vi "Speed.vi"(8 "error in":errorcluster, 11 "Parrot in":refnum<class "Parrot.lvclass">) -> (0 "error out":errorcluster, 2 "Speed":dbl, 3 "Parrot out":refnum<class "Parrot.lvclass">)   [LabVIEW 2020, in "Parrot.lvclass"]
uses:
  Parrot.lvclass
  Parrot.lvclass/Parrot.ctl
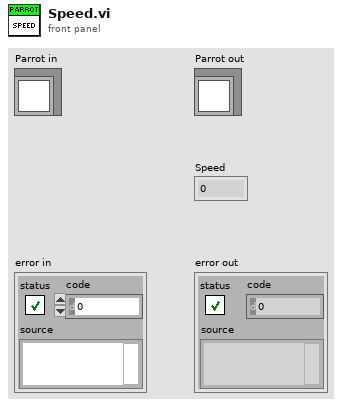
[diagram p1: front panel]
types:
  T1 = typedef "Parrot.lvclass/Parrot Type.ctl" = enum16{"European", "African", "Norwegian Blue"}
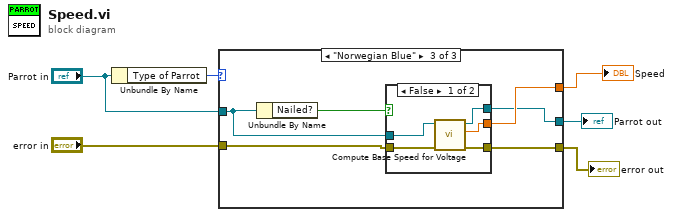
[diagram p0: block diagram]
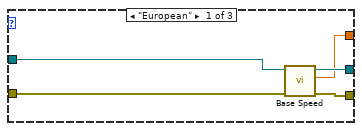
[diagram p2: hidden frame]
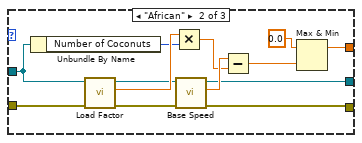
[diagram p3: hidden frame]
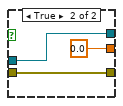
[diagram p4: hidden frame]
diagram:
  n1 = Unbundle By Name("Parrot in") -> ("Type of Parrot"=w4:T1)
  n2 = case shown="\"Norwegian Blue\"" w4 {
    tunnel: "Parrot in" -> [w9 w16 w26]
    tunnel: [w8 w14 w25] -> w2
    tunnel: [w7 w13 w27] -> w1
    tunnel: "error in" -> [w11 w24 w30]
    tunnel: [w10 w22 w29] -> w5
    frame "European" {
      n3 = call "Base Speed.vi"("error in"=w11, "Parrot in"=w9) -> ("error out"=w10:errorcluster, "Base Speed"=w7:dbl, "Parrot out"=w8:refnum<class "Parrot.lvclass">)  [unwired: 7 in]
    }
    frame "African" {
      n4 = Unbundle By Name(w16) -> ("Number of Coconuts"=w17:i32)
      n5 = call "Load Factor.vi"("error in"=w24, "Parrot in"=w16) -> ("error out"=w23:errorcluster, "Load Factor"=w19:dbl, "Parrot out"=w15:refnum<class "Parrot.lvclass">)  [unwired: 7 in]
      n6 = Multiply(x=w19, y=w17) -> (x*y=w18:dbl)
      n7 = call "Base Speed.vi"("error in"=w23, "Parrot in"=w15) -> ("error out"=w22:errorcluster, "Base Speed"=w20:dbl, "Parrot out"=w14:refnum<class "Parrot.lvclass">)  [unwired: 7 in]
      n8 = Subtract(x=w20, y=w18) -> (x-y=w12:dbl)
      n9 = Max & Min(x=0.0, y=w12) -> (max(x,y)=w13:dbl)  [unwired: 1 out]
    }
    frame "Norwegian Blue" {
      n10 = Unbundle By Name(w26) -> ("Nailed?"=w28:bool)
      n11 = case shown="False" w28 {
        tunnel: [w33 0.0] -> w27
        tunnel: w26 -> [w32 w36]
        tunnel: [w31 w36] -> w25
        tunnel: [w34 w38] -> w29
        tunnel: w30 -> [w35 w38]
        frame False {
          n12 = call "Compute Base Speed for Voltage.vi"("error in"=w35, "Parrot in"=w32) -> ("error out"=w34:errorcluster, "Adjusted Base Speed"=w33:dbl, "Parrot out"=w31:refnum<class "Parrot.lvclass">)  [unwired: 7 in]
        }
        frame True {
        }
      }
    }
  }
  "error out" <- w5
  "Parrot out" <- w2
  "Speed" <- w1
